vi "Setup.vi"(8 "error in (no error)":errorcluster, 11 "LUnit Test Read File In":refnum<class "Test Read File.lvclass">) -> (0 "error out":errorcluster, 3 "LUnit Test Read File Out":refnum<class "Test Read File.lvclass">)   [LabVIEW 2019, in "Test Read File.lvclass"]
doc: "Setup method called by the testing framework to set up test fixture before each test method is called."
uses:
  Test Read File.lvclass
  Test Read File.lvclass/Test Read File.ctl
  <vilib>/Astemes/LUnit/Test Case.lvclass
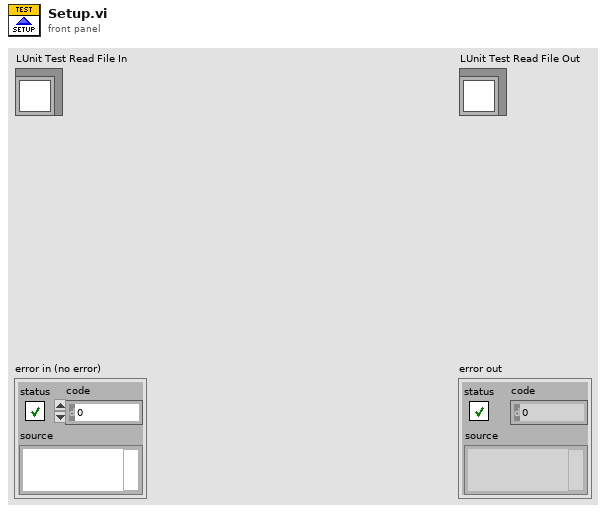
[diagram p1: front panel]
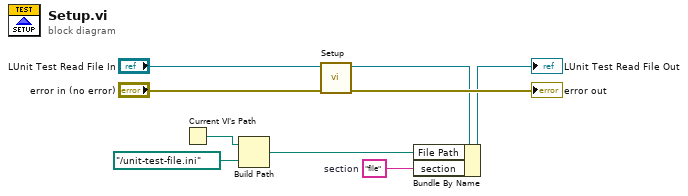
[diagram p0: block diagram]
diagram:
  w1 = "file"  # section
  n1 = Current VI's Path() -> (path=w5:path)
  n2 = Build Path(base path=w5, name or relative path=path "../unit-test-file.ini") -> (appended path=w2:path)
  n3 = call-parent "Setup.vi"("error in (no error)"="error in (no error)", "LUnit Test Case In"="LUnit Test Read File In") -> ("error out"=→"error out":errorcluster, "LUnit Test Case Out"=w8:refnum<class "Test Read File.lvclass">)  [unwired: 8 in]
  n4 = Bundle By Name(cluster=w8, "File Path"=w2, "section"=w1) -> (→"LUnit Test Read File Out":refnum<class "Test Read File.lvclass">)
